vi "Draw Navigation Picture.vi"(8 "Offset":T1, 9 "UI Selections":T2, 10 "Pane Details":T3[](array[typedef]), 11 "Splitter Details":T4[](array[typedef])) -> (3 "Navigation Picture":picture)   [LabVIEW 2018]
uses:
  Typedefs/Splitter Details--Cluster.ctl
  Typedefs/Pane Details--Cluster.ctl
  Typedefs/UI Selections--Cluster.ctl
  Typedefs/Point--Cluster.ctl
  Typedefs/Selection Colors--Cluster.ctl
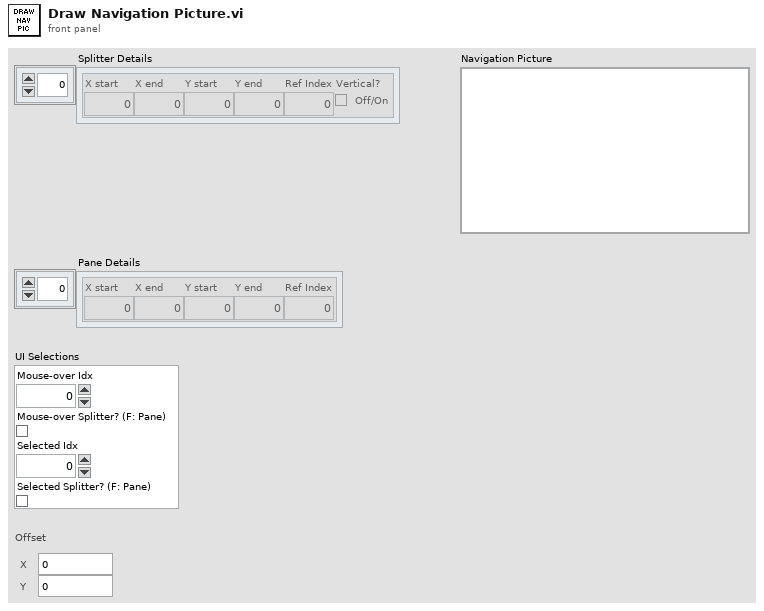
[diagram p1: front panel]
types:
  T1 = typedef "Point--Cluster.ctl" = cluster{"Horizontal":i32, "Vertical":i32}
  T2 = typedef "UI Selections--Cluster.ctl" = cluster{"Mouse-over Idx":i32, "Mouse-over Splitter? (F: Pane)":bool, "Selected Idx":i32, "Selected Splitter? (F: Pane)":bool}
  T3 = typedef "Pane Details--Cluster.ctl" = cluster{"X start":i32, "X end":i32, "Y start":i32, "Y end":i32, "Ref Index":i32}
  T4 = typedef "Splitter Details--Cluster.ctl" = cluster{"X start":i32, "X end":i32, "Y start":i32, "Y end":i32, "Ref Index":i32, "Vertical?":bool}
  T5 = cluster{"left":i16, "top":i16, "right":i16, "bottom":i16}
  T6 = typedef "Selection Colors--Cluster.ctl" = cluster{"Normal":u32, "Mouse-over":u32, "Selected":u32}
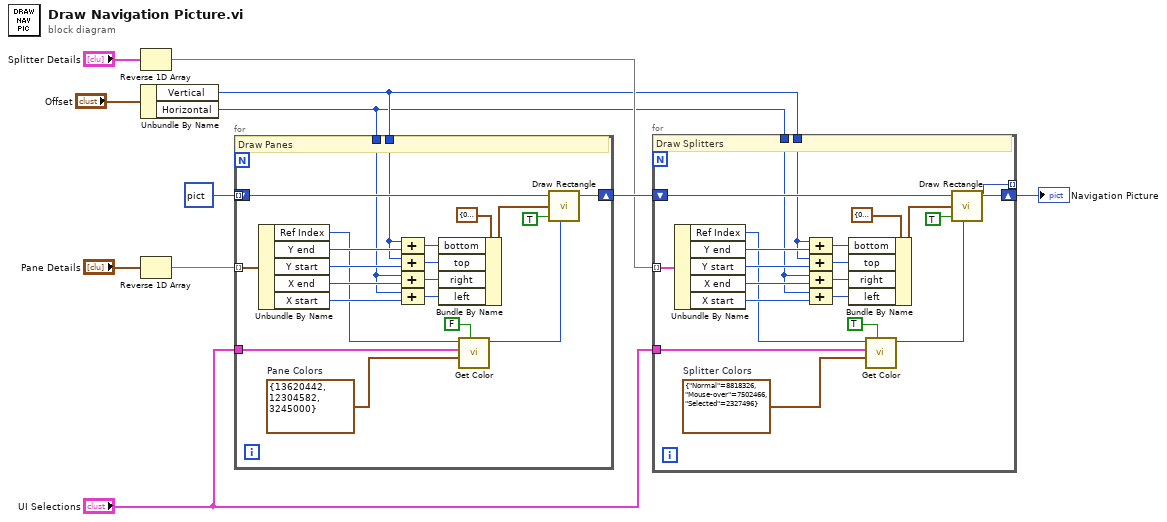
[diagram p0: block diagram]
diagram:
  n1 = Reverse 1D Array(array="Splitter Details") -> (reversed array=w4:T4[])
  n2 = Unbundle By Name("Offset") -> ("Vertical"=w2:i32, "Horizontal"=w1:i32)
  n3 = Reverse 1D Array(array="Pane Details") -> (reversed array=w5:T3[])
  n4 = for {
    shift-right: [w23] -> w7
    shift-left: picture data[5B] ("new picture") -> [w32]
    tunnel: w5 -> [w24] mode=indexing
    tunnel: [w23] -> _ mode=indexing
    tunnel: "UI Selections" -> [w20]
    tunnel: w1 -> [w13]
    tunnel: w2 -> [w12]
    w19 = T6 {"Normal"=13620442, "Mouse-over"=12304582, "Selected"=3245000}  # Pane Colors
    # "Draw Panes"
    n5 = Unbundle By Name(w24) -> ("Ref Index"=w22:i32, "Y end"=w28:i32, "Y start"=w27:i32, "X end"=w26:i32, "X start"=w25:i32)
    n6 = Compound Arithmetic op=ADD(w12, w28) -> (w16:i32)
    n7 = Compound Arithmetic op=ADD(w12, w27) -> (w17:i32)
    n8 = Compound Arithmetic op=ADD(w13, w26) -> (w15:i32)
    n9 = Compound Arithmetic op=ADD(w13, w25) -> (w14:i32)
    n10 = Bundle By Name(cluster=T5 {"left"=0, "top"=0, "right"=0, "bottom"=0} ("rect"), "bottom"=w16, "top"=w17, "right"=w15, "left"=w14) -> (w29:T5)
    n11 = call "Get Color.vi"("Splitter? (F: Pane)"=FALSE, "Pane Colors"=w19, "UI Selections"=w20, "Item Index"=w22) -> ("Color"=w21:u32)  [unwired: 7 in]
    n12 = call <vilib>:"Draw Rectangle.vi"("picture"=w32, "rect"=w29, "fill?(F)"=TRUE, "color(black)"=w21) -> ("new picture"=w23:picture)  [unwired: 5 in]
  }
  n13 = for {
    tunnel: w4 -> [w45] mode=indexing
    shift-right: [w53] -> w6
    shift-left: w7 -> [w44]
    tunnel: [w44] -> _ mode=indexing
    tunnel: "UI Selections" -> [w41]
    tunnel: w2 -> [w34]
    tunnel: w1 -> [w33]
    w40 = T6 {"Normal"=8818326, "Mouse-over"=7502466, "Selected"=2327496}  # Splitter Colors
    # "Draw Splitters"
    n14 = Unbundle By Name(w45) -> ("Ref Index"=w43:i32, "Y end"=w49:i32, "Y start"=w48:i32, "X end"=w47:i32, "X start"=w46:i32)
    n15 = Compound Arithmetic op=ADD(w34, w49) -> (w38:i32)
    n16 = Compound Arithmetic op=ADD(w34, w48) -> (w37:i32)
    n17 = Compound Arithmetic op=ADD(w33, w47) -> (w36:i32)
    n18 = Compound Arithmetic op=ADD(w33, w46) -> (w35:i32)
    n19 = Bundle By Name(cluster=T5 {"left"=0, "top"=0, "right"=0, "bottom"=0} ("rect"), "bottom"=w38, "top"=w37, "right"=w36, "left"=w35) -> (w50:T5)
    n20 = call "Get Color.vi"("Splitter? (F: Pane)"=TRUE, "Pane Colors"=w40, "UI Selections"=w41, "Item Index"=w43) -> ("Color"=w42:u32)  [unwired: 7 in]
    n21 = call <vilib>:"Draw Rectangle.vi"("picture"=w44, "rect"=w50, "fill?(F)"=TRUE, "color(black)"=w42) -> ("new picture"=w53:picture)  [unwired: 5 in]
  }
  "Navigation Picture" <- w6
